vi "testProjectLibrary.vi"() -> (0 "error out":errorcluster)   [LabVIEW 2019, in "TestSuiteTest.lvlib" / "Create.lvlib"]
uses:
  Create.lvlib
  cd5b1fa9-69d3-4d24-ae9c-3424e7998d9a.vi
  Constraint/IsEqual/IsEqual.lvclass
  TestSuite/TestSuite.lvclass
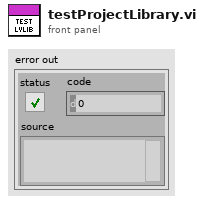
[diagram p1: front panel]
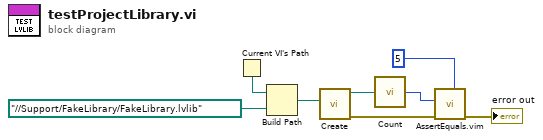
[diagram p0: block diagram]
diagram:
  n1 = Current VI's Path() -> (path=w2:path)
  n2 = Build Path(base path=w2, name or relative path=path "../../Support/FakeLibrary/FakeLibrary.lvlib" ("Path")) -> (appended path=w3:path)
  n3 = call "Create.vi"("Path"=w3) -> ("error out"=w6:errorcluster, "TestSuite"=w8:refnum<class "TestSuite.lvclass">)  [unwired: 9 in]
  n4 = call "Count.vi"("TestSuite In"=w8) -> ("Count"=w7:i32)
  n5 = call "AssertEquals.vim"("Expected"=5 ("Count"), "error in (no error)"=w6, "Actual"=w7) -> ("error out"=→"error out":errorcluster)  [unwired: 8 in]
